vi "RT_VS50_Dynamics_DLR_v2.vi"() -> ()   [LabVIEW 2017]
uses:
  <vilib>/Platform/TimedLoop/XDataNode/timing_clust.ctl
  <vilib>/Platform/TimedLoop/XDataNode/nitl_modes.ctl
  <vilib>/Platform/TimedLoop/XDataNode/wakeup.ctl
  <vilib>/Analysis/coordinate.llb/Euler Rotation Order.ctl
  <vilib>/Analysis/baseanly.llb/Real A x B.vi
  <vilib>/Utility/file.llb/Read Delimited Spreadsheet (DBL).vi
  <vilib>/FPGAPlugInAG/Dynamic/niLvFpga_Close_Dynamic.vi
  <vilib>/Analysis/Matrix/Numeric/Conversions/Array To Matrix - RA2.vi
  <vilib>/Analysis/Matrix/Numeric/Conversions/Array To Matrix - RA.vi
  <vilib>/Analysis/Matrix/Numeric/Conversions/Matrix To Array - RM.vi
  <vilib>/platform/TimedLoop/XDataNode/XDataNode.xnode
  <vilib>/rvi/interface/nirviCloseFPGA/nirviCloseFPGA.xnode
  <vilib>/Platform/TimedLoop/XDataNode/XDNodeRunTimeDep.lvlib
  <vilib>/Analysis/Matrix/NI_Matrix.lvlib
  <vilib>/Analysis/NI_AALBase.lvlib
  <vilib>/Analysis/NI_AALPro.lvlib
panel:
  out "all rows":dbl[][](array[numeric]) format="%.9g"
  out "Math_OUT":dbl[](array[numeric])
  out "Velocity Mach":dbl
  out "latd(i) [º]":dbl
  out "lon(i) [º]":dbl
  out "acc_b":dbl[](array[numeric])
  out "SIM_Running 2":bool
  in  "Constant wind [m/s]":dbl format="%#_13g"
  out "Data 4":dbl[][](array[numeric])
  out "Data 3":dbl[][](array[numeric])
  in  "Wind_File":i32=1
  out "Data 2":dbl[][](array[numeric])
  out "TVA_Data CRC Fault":bool
  out "TVA_Address CRC Fault":bool
  out "Log":i64
  out "spreadsheet string":string
  in  "UTC format":bool
  out "appended path":path
  out "concatenated string":string
  out "SIM_Running":bool
  in  "stop RT":bool
  out "DMARS Write":i64
  out "TVA read":i64
  out "TVA_data":dbl[](array[numeric])
  out "bad iteration":bool
  out "Sim_Time":dbl
  out "string_DMARS":string
  out "lon(i) [rad]":dbl
  out "Euler Angles [rad]":dbl[](array[numeric])
  out "Euler Angles [º]":dbl[](array[numeric])
  out "M_beta":dbl
  out "M_alpha":dbl
  out "TVA_cmd [rad]":dbl[](array[numeric])
  out "Sref [m^2]":dbl
  out "MAd [Nm]":dbl[](array[numeric])
  out "MA_f [Nm]":dbl[](array[numeric])
  out "act_b":dbl[](array[numeric])
  out "p(i) [m]":dbl[](array[numeric])
  out "MFE_b":dbl[](array[numeric])
  out "alt(i) [m]":dbl
  out "latd(i) [rad]":dbl
  out "W_b(i) [º/s]":dbl[](array[numeric])
  out "q(i)":dbl[](array[numeric])
  out "W(i)":dbl[](array[numeric])
  out "V(i) [m/s]":dbl[](array[numeric])
  out "W(i+1)":dbl[](array[numeric])
  out "q(i+1)":dbl[](array[numeric])
  out "t [s]":dbl
  out "dt[s]":dbl
  out "ang_acc [rad/s^2]":dbl[](array[numeric])
  out "acc [m/s^2]":dbl[](array[numeric])
  out "MFA [Nm]":dbl[](array[numeric])
  out "MFE [Nm]":dbl[](array[numeric])
  out "Mco [Nm]":dbl[](array[numeric])
  out "Fco [N]":dbl[](array[numeric])
  out "FA [N]":dbl[](array[numeric])
  out "FG_b [N]":dbl[](array[numeric])
  out "FG [N]":dbl[](array[numeric])
  out "FE [N]":dbl[](array[numeric])
  out "FE_b [N]":dbl[](array[numeric])
  out "AoA_yaw [rad]":dbl
  out "AoA_pitch [rad]":dbl
  out "Iteration Duration [us]":i64(graph)
  out "Patm [Pa]":dbl
  out "Pdin [Pa]":dbl
  out "Nzl_S [m^2]":dbl
  out "Data":dbl[][](array[numeric])
  # "Time"
  # "TVA command"
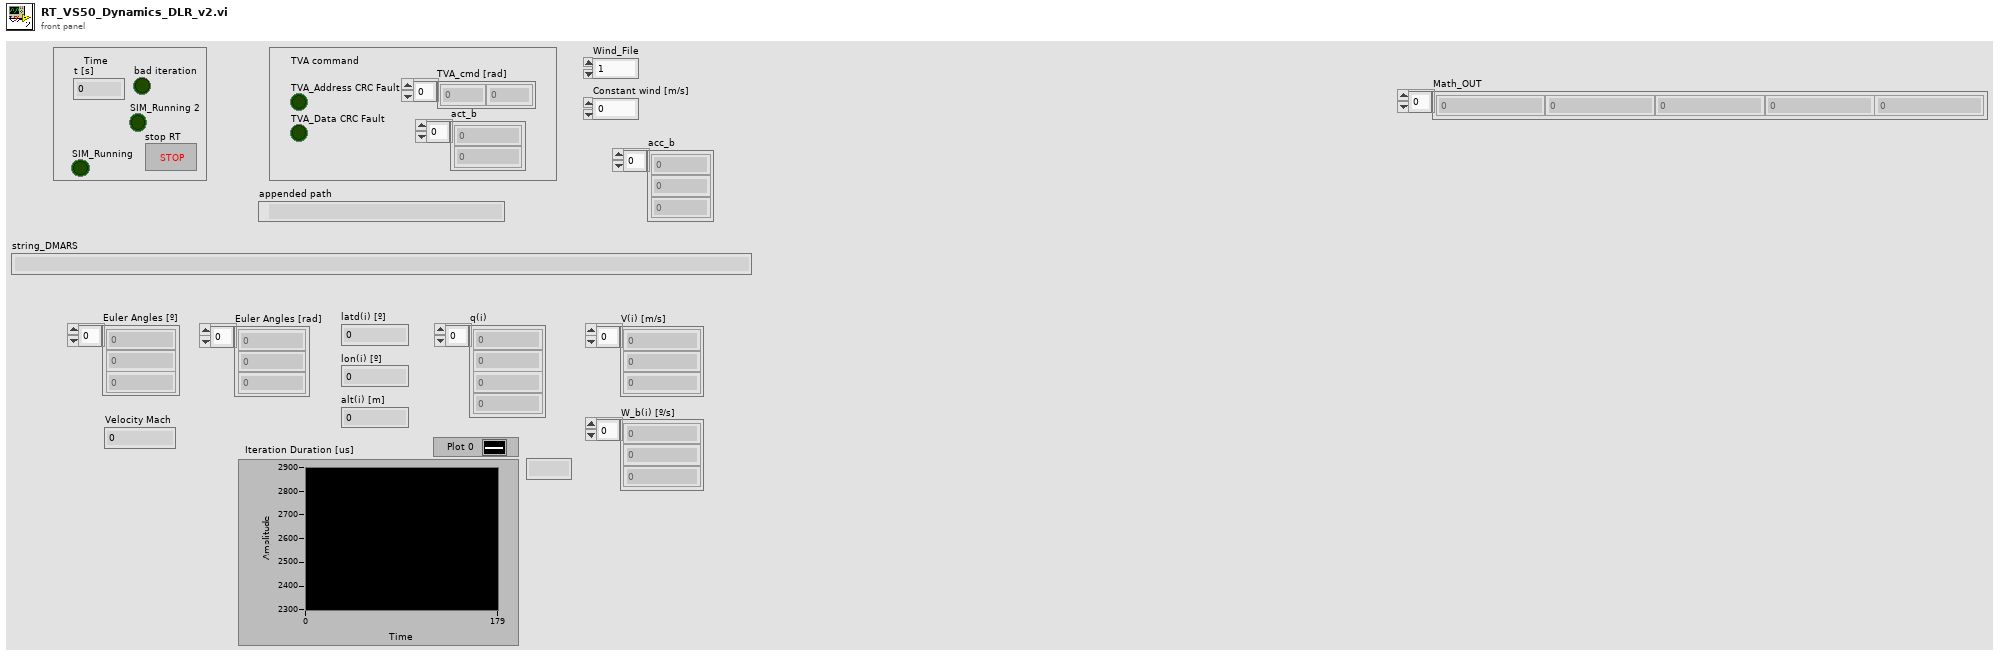
[diagram p1: front panel]
types:
  T1 = enum16{"open", "replace", "create", "open or create", "replace or create", "replace or create with confirmation"}
  T2 = typedef "XDNodeRunTimeDep.lvlib/timing_clust.ctl" = cluster{"Expected End [f-1]":u64, "Actual End [f-1]":u64, "Finished Late? [f-1]":bool, "Expected End [i-1]":u64, "Actual End [i-1]":u64, "Finished Late? [i-1]":bool, "Expected Start [i]":u64, "Actual Start [i]":u64, "Expected Start [f]":u64, "Actual Start [f]":u64, "Source Name":string, "Structure Name":string, "Period":i64, "Deadline":i64, "Offset":i64, "Start":i64, "Priority":i32, "Timeout":i32, "Mode":T3, "Wakeup Reason":T4, "Error":errorcluster, "Source Type":string, "Secondary Source Type":string, "Global End Time":u64, "Global Start Time":u64, "Frame Duration":u64, "Iteration Duration":u64, "Assigned CPU":i32, "I/O Scan Engine Mode":u32}
  T3 = typedef "XDNodeRunTimeDep.lvlib/nitl_modes.ctl" = enum32{"No Change", "Process missed periods, maintain original phase", "Discard missed periods, maintain original phase", "Process missed periods, ignore original phase", "Discard missed periods, ignore original phase"}
  T4 = typedef "XDNodeRunTimeDep.lvlib/wakeup.ctl" = enum32{"Normal", "Aborted", "Asynchronous wakeup", "Timing source error", "Timed loop error", "Timeout"}
  T5 = typedef "NI_AALPro.lvlib/Euler Rotation Order.ctl" = u16
  T6 = typedef "NI_Matrix.lvlib/RealMatrix.ctl" = dbl[][]
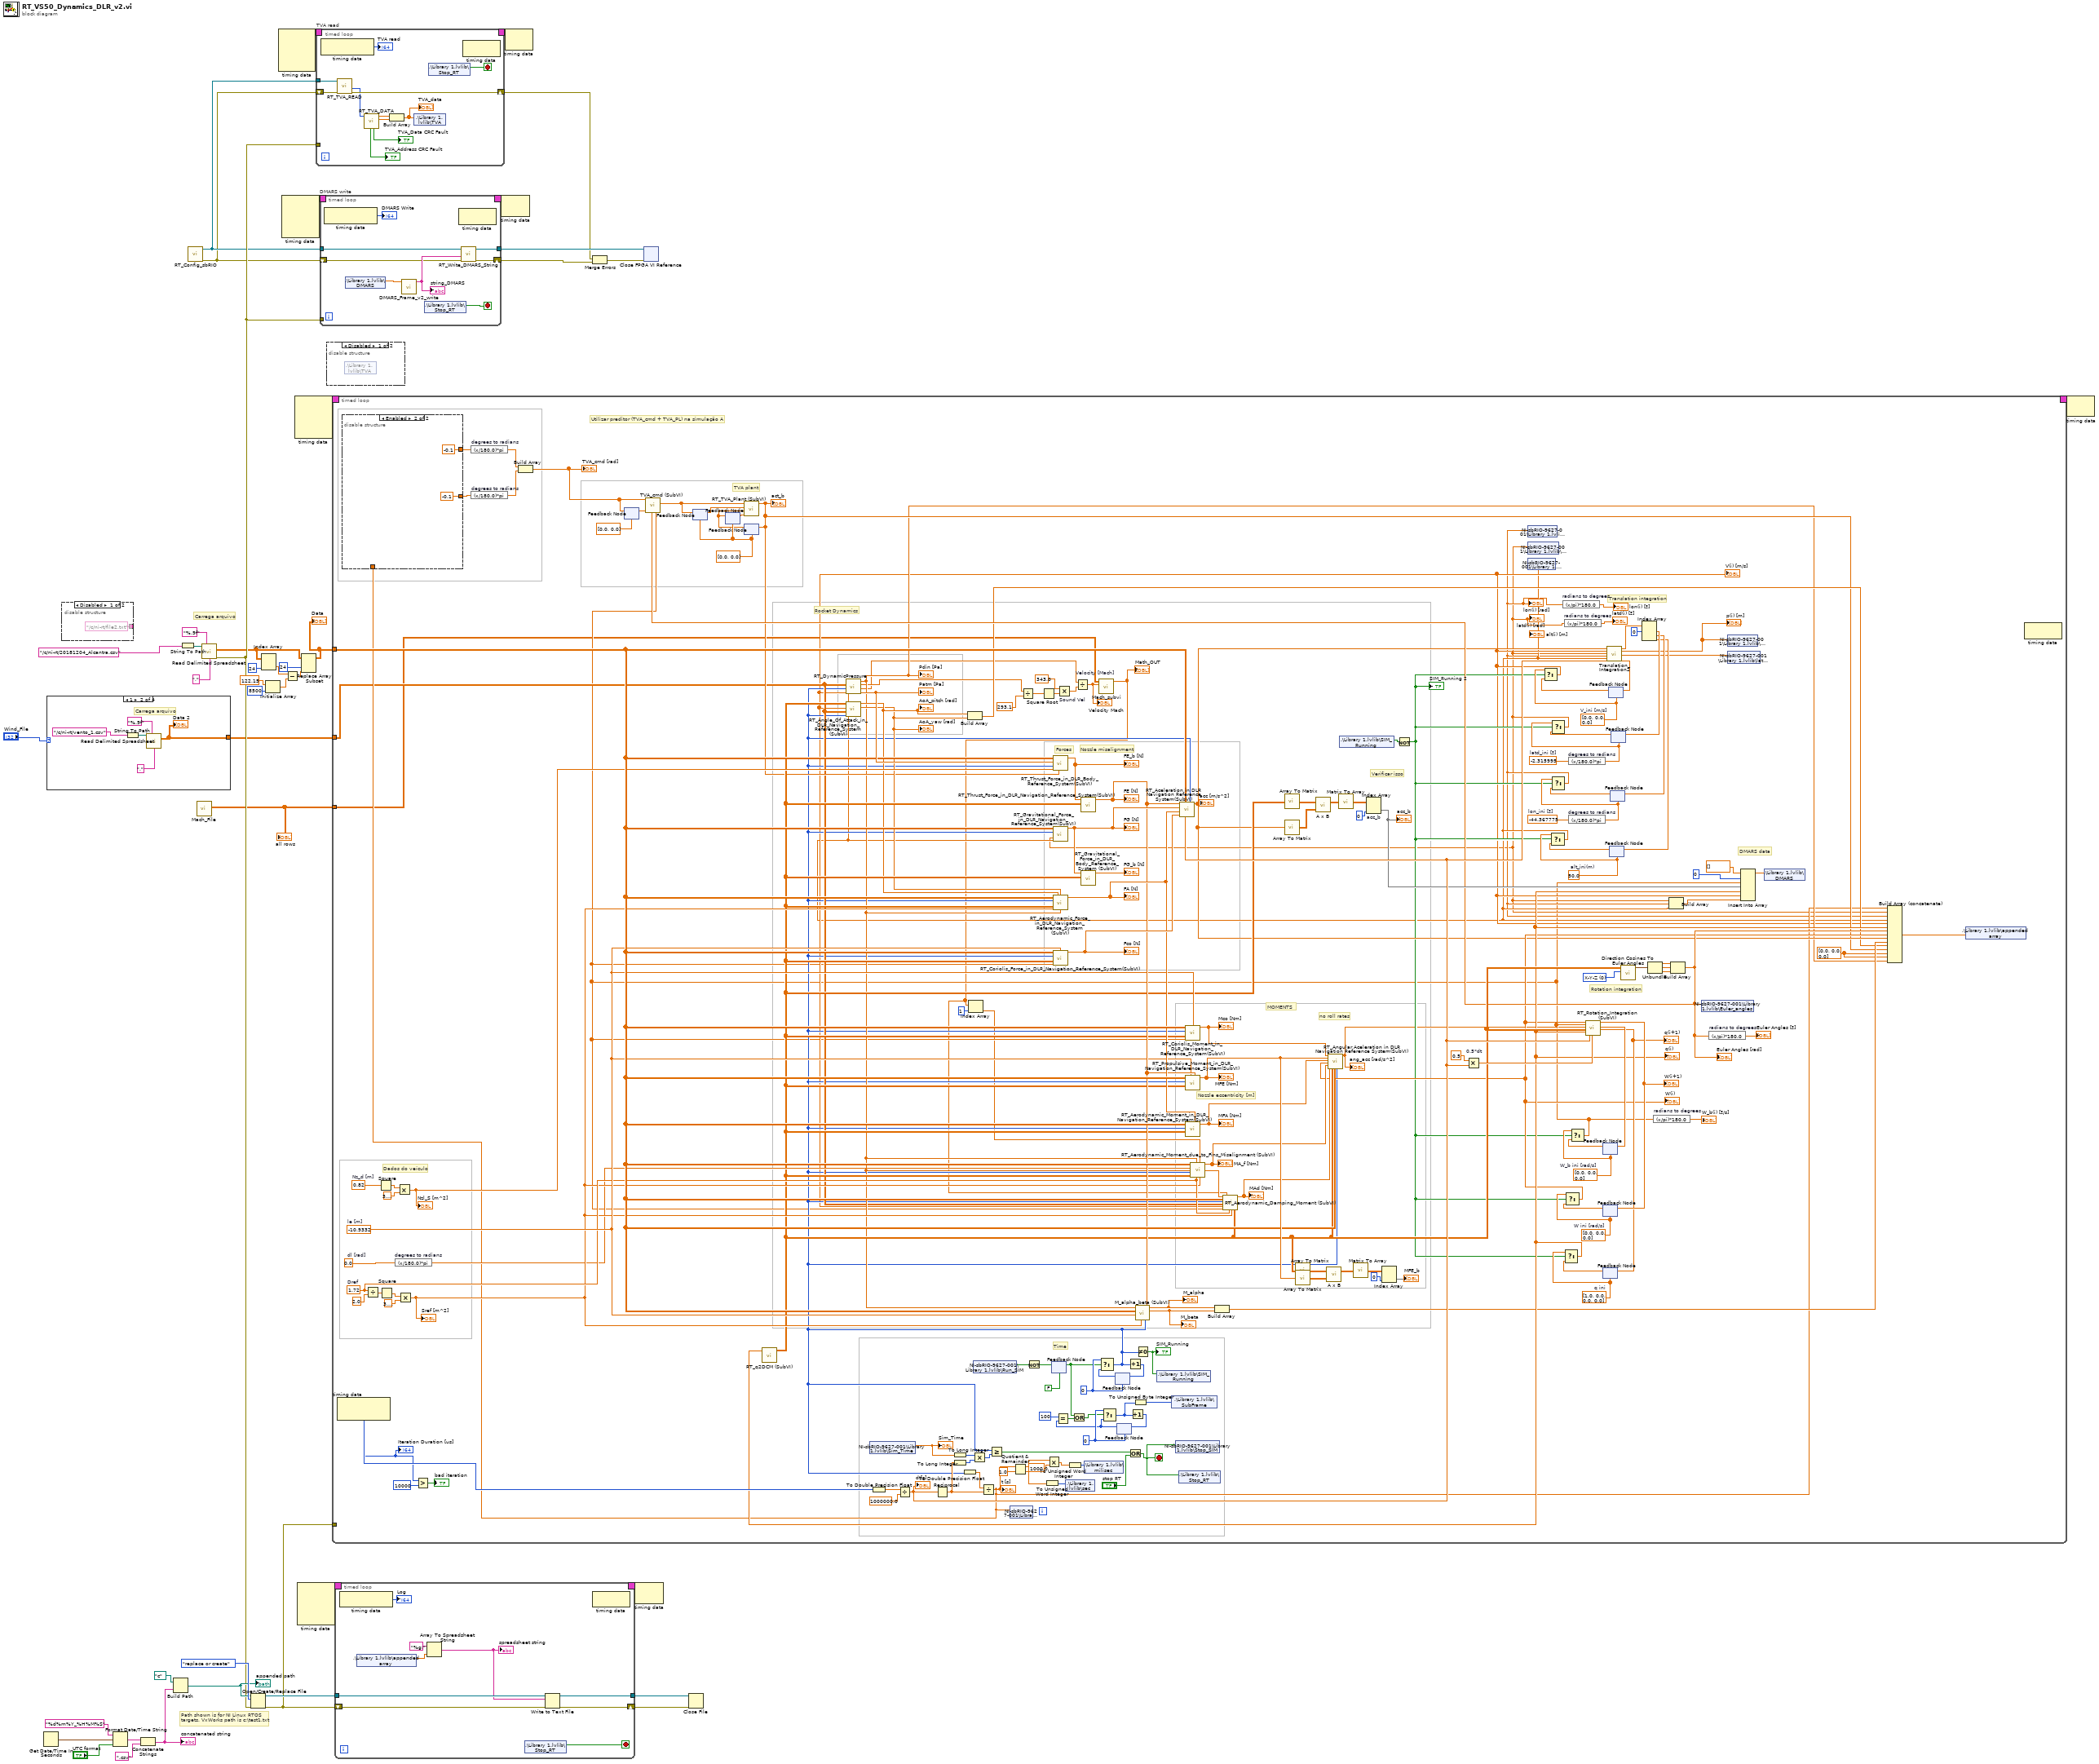
[diagram p0: block diagram]
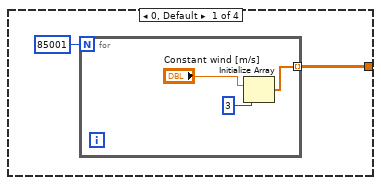
[diagram p4: hidden frame]
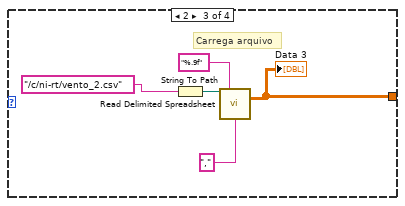
[diagram p5: hidden frame]
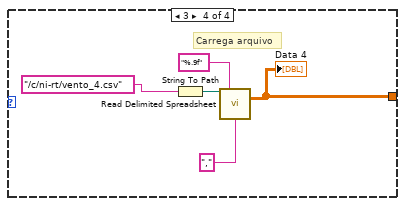
[diagram p6: hidden frame]
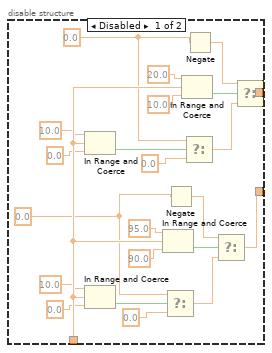
[diagram p7: hidden frame]
diagram:
  # "Path shown is for NI Linux RTOS\ntargets. VxWorks path is c:\\test1.txt"
  # "Carrega arquivo"
  n1 = Get Date/Time In Seconds() -> (seconds since 1Jan1904=w28:timestamp)
  n2 = case shown="1" "Wind_File" {
    tunnel: [w45 w50 w55 w60] -> w12
    frame 0, Default {
      n3 = for {
        N: 85001 -> [_]
        tunnel: [w47] -> w45 mode=indexing
        n4 = Initialize Array("Constant wind [m/s]", 3 ("dimension size")) -> (w47:dbl[])
      }
    }
    frame 1 {
      # "Carrega arquivo"
      n5 = String To Path(string="/c/ni-rt/vento_1.csv") -> (path=w52:path)
      n6 = call-poly <vilib>:"Read Delimited Spreadsheet.vi"("file path (dialog if empty)"=w52, "format (%.3f)"="%.9f", "delimiter (\\t)"="," ("delimiter (\\t)")) -> ("all rows"=w50:dbl[][])  [unwired: 7 in, 5 out]
      "Data 2" <- w50
    }
    frame 2 {
      # "Carrega arquivo"
      n7 = String To Path(string="/c/ni-rt/vento_2.csv") -> (path=w57:path)
      n8 = call-poly <vilib>:"Read Delimited Spreadsheet.vi"("file path (dialog if empty)"=w57, "format (%.3f)"="%.9f", "delimiter (\\t)"="," ("delimiter (\\t)")) -> ("all rows"=w55:dbl[][])  [unwired: 7 in, 5 out]
      "Data 3" <- w55
    }
    frame 3 {
      # "Carrega arquivo"
      n9 = String To Path(string="/c/ni-rt/vento_4.csv") -> (path=w62:path)
      n10 = call-poly <vilib>:"Read Delimited Spreadsheet.vi"("file path (dialog if empty)"=w62, "format (%.3f)"="%.9f", "delimiter (\\t)"="," ("delimiter (\\t)")) -> ("all rows"=w60:dbl[][])  [unwired: 7 in, 5 out]
      "Data 4" <- w60
    }
  }
  n11 = disable-structure shown="Disabled" {
    disable-tunnel: ["/c/ni-rt/file2.txt" _] -> _
    frame Disabled {
    }
    frame Enabled {
    }
  }
  n12 = Format Date/Time String(time format string (%c)="%d%m%Y_%H%M%S", seconds (now)=w28, UTC format="UTC format") -> (date/time string=w27:string)
  n13 = Concatenate Strings(w27, ".csv" ("string")) -> (w33:string)
  "concatenated string" <- w33
  n14 = Build Path(base path=path "c:/" ("file path (use dialog)"), name or relative path=w33) -> (appended path=w31:path)
  "appended path" <- w31
  n15 = String To Path(string="/c/ni-rt/20181204_Alcantra.csv") -> (path=w44:path)
  n16 = call "RT_Config_sbRIO.vi"() -> ("error out"=w17:errorcluster, "FPGA VI  Out"=w18:refnum<k20>)  [unwired: 10 in]
  n17 = call "Mach_File.vi"() -> ("all rows"=w1:dbl[][])  [unwired: 10 in, 1 out]
  "all rows" <- w1
  n18 = call-poly <vilib>:"Read Delimited Spreadsheet.vi"("file path (dialog if empty)"=w44, "format (%.3f)"="%.9f", "delimiter (\\t)"="," ("delimiter (\\t)")) -> ("all rows"=w3:dbl[][], "error out"=w25:errorcluster)  [unwired: 7 in, 4 out]
  n19 = Open/Create/Replace File(file path (use dialog)=w31, error in=w25, operation (0:open)=T1."replace or create") -> (refnum out=w36:refnum<file>, error out=w24:errorcluster)  [unwired: 3 in, 1 out]
  n20 = Index Array(array=w3, index (col)=24 ("disabled index (col)")) -> (element=w9:dbl[])  [unwired: 1 in]
  n21 = Initialize Array(122.15 ("element"), 8500 ("dimension size")) -> (w6:dbl[])
  n22 = node-c288() -> (w21:T2)  [unwired: 4 in]
  n23 = node-c288() -> (w23:T2)  [unwired: 4 in]
  n24 = Subtract(x=w9, y=w6) -> (x-y=w5:dbl[])
  n25 = node-c288() -> (w41:T2)  [unwired: 4 in]
  n26 = node-c288() -> (w39:T2)  [unwired: 4 in]
  n27 = Replace Array Subset(array=w3, new element=w5, index (col)=24 ("disabled index (col)")) -> (w2:dbl[][])  [unwired: 1 in]
  "Data" <- w2
  n28 = timed-loop "TVA read" {
    timing: w21 -> [_]
    timing-out: [_] -> w20
    tunnel: w18 -> [w76]
    shift-right: [w73] -> w15
    shift-left: w17 -> [w75]
    tunnel: w25 -> [_]
    stop <- w74 stop-if-true
    n29 = node-c288() -> (→"TVA read":i64)  [unwired: 1 in]
    n30 = call "RT_TVA_READ.vi"("error in (no error)"=w75, "FPGA VI  IN"=w76) -> ("error out"=w73:errorcluster, "Data"=w72:u64[])  [unwired: 7 in, 1 out]
    n31 = call "RT_TVA_DATA.vi"("TVA_Data"=w72) -> ("Yaw Angle"=w70:dbl, "Pitch Angle"=w71:dbl, "Data CRC Fault"=→"TVA_Data CRC Fault":bool, "Address CRC Fault"=→"TVA_Address CRC Fault":bool)  [unwired: 5 in, 2 out]
    n32 = Build Array(w71, w70) -> (w69:dbl[])
    "TVA_data" <- w69
    n33 = shared-variable ".\\Library 1.lvlib\\TVA"(w69) -> ()  [unwired: 1 in, 1 out]
    n34 = shared-variable ".\\Library 1.lvlib\\Stop_RT"() -> (w74:bool)  [unwired: 1 in, 1 out]
    n35 = node-c288() -> ()  [unwired: 1 in, 1 out]
  }
  n36 = timed-loop "DMARS write" {
    timing: w23 -> [_]
    timing-out: [_] -> w22
    tunnel: w25 -> [_]
    tunnel: w18 -> [w85]
    tunnel: [w83] -> w19
    shift-right: [w82] -> w14
    shift-left: w17 -> [w84]
    stop <- w87 stop-if-true
    n37 = node-c288() -> (→"DMARS Write":i64)  [unwired: 1 in]
    n38 = shared-variable ".\\Library 1.lvlib\\DMARS"() -> (w81:dbl[])  [unwired: 1 in, 1 out]
    n39 = call "DMARS_Frame_v2_write.vi"("DMARS"=w81) -> ("string_Out"=w86:string)  [unwired: 10 in]
    "string_DMARS" <- w86
    n40 = shared-variable ".\\Library 1.lvlib\\Stop_RT"() -> (w87:bool)  [unwired: 1 in, 1 out]
    n41 = node-c288() -> ()  [unwired: 1 in, 1 out]
    n42 = call "RT_Write_DMARS_String.vi"("error in (no error)"=w84, "String"=w86, "FPGA VI  IN"=w85) -> ("error out"=w82:errorcluster, "FPGA VI  Out"=w83:refnum<k20>)  [unwired: 7 in]
  }
  n43 = disable-structure shown="Disabled" {
    frame Disabled {
      n44 = shared-variable ".\\Library 1.lvlib\\TVA"() -> ()  [unwired: 1 in, 2 out]
    }
    frame Enabled {
    }
  }
  n45 = timed-loop {
    timing: w41 -> [_]
    timing-out: [_] -> w40
    tunnel: w2 -> [w234]
    tunnel: w24 -> [_]
    tunnel: w12 -> [w131]
    tunnel: w1 -> [w99]
    stop <- w142 stop-if-true
    w95 = dbl[] [0.0, 0.0] ("TVA_b")
    w217 = -44.367775  # lon_ini [º]
    w216 = -2.315995  # latd_ini [º]
    w123 = 0 ("x")
    w147 = dbl[] [0.0, 0.0, 0.0] ("array")
    w175 = 0 ("x")
    w189 = T5 0 items=["X-Y-Z", "X-Z-Y", "Y-X-Z", "Y-Z-X", "Z-X-Y", "Z-Y-X", "X-Y-X", "X-Z-X", "Y-X-Y", "Y-Z-Y", "Z-X-Z", "Z-Y-Z"] ("rotation order")
    w206 = 1.72  # Dref
    w195 = 0.0  # dl [rad]
    w211 = 0.82  # Nz_d [m]
    w207 = -10.9332  # le [m]
    w162 = dbl[] [0.0, 0.0, 0.0]  # W_b ini [rad/s]
    w168 = dbl[] [0.0, 0.0, 0.0]  # V_ini [m/s]
    w164 = 50.0  # alt_ini(m)
    w160 = dbl[] [0.0, 0.0, 0.0]  # W ini [rad/s]
    w158 = dbl[] [1.0, 0.0, 0.0, 0.0]  # q ini
    # "no roll rates"
    # "TVA plant"
    # "Nozzle eccentricity [m]"
    # "Nozzle misalignment"
    # "DMARS data"
    # "Rotation integration"
    # "Translation integration"
    # "Utilizar preditor (TVA_cmd + TVA_PL) na simulação A"
    # "Verificar isso"
    # "Rocket Dynamics"
    # "Time"
    # "Dados do veículo"
    # "MOMENTS"
    # "Forces"
    n46 = node-c288() -> (w193:i64, w254:i64)  [unwired: 1 in]
    "Iteration Duration [us]" <- w193
    n47 = Divide(x=w206, y=2.0) -> (x/y=w215:dbl)
    n48 = Square(x=w211) -> (x^2=w209:dbl)
    n49 = Square(x=w215) -> (x^2=w214:dbl)
    n50 = expression code="(x/180.0)*pi" "degrees to radians"(w195) -> (w194:dbl)
    n51 = Multiply(x=w209, y=3.141592653589793) -> (x*y=w208:dbl)
    "Nzl_S [m^2]" <- w208
    n52 = Multiply(x=w214, y=3.141592653589793) -> (x*y=w205:dbl)
    "Sref [m^2]" <- w205
    n53 = Greater?(x=w193, y=i64 10000) -> (0:→"bad iteration":bool)
    n54 = feedback #1(dbl[] [0.0, 0.0] ("TVA_cmd")) -> (w190:dbl[])
    n55 = feedback #2(w95) -> (w94:dbl[])
    n56 = feedback #3(w95) -> (w92:dbl[])
    n57 = feedback #4(w95) -> (w93:dbl[])
    n58 = feedback-in #3(w93) -> ()
    n59 = shared-variable "NI-sbRIO-9627-001\\Library 1.lvlib\\Sim_Time"() -> (w196:dbl)  [unwired: 1 in, 1 out]
    "Sim_Time" <- w196
    n60 = To Double Precision Float(number=w254) -> (double precision float=w253:dbl)
    n61 = Divide(x=w253, y=1000000.0) -> (x/y=w223:dbl)
    "dt[s]" <- w223
    n62 = Reciprocal(x=w223) -> (1/x=w250:dbl)
    n63 = To Long Integer(number=w196) -> (32bit integer=w197:i32)
    n64 = To Long Integer(number=w250) -> (32bit integer=w251:i32)
    n65 = Multiply(x=w197, y=w251) -> (x*y=w259:i32)
    n66 = shared-variable "NI-sbRIO-9627-001\\Library 1.lvlib\\Run_SIM"() -> (w172:bool)  [unwired: 1 in, 1 out]
    n67 = Not(x=w172) -> (.not. x?=w143:bool)
    n68 = feedback-in #5(w143) -> ()
    n69 = feedback #5(FALSE) -> (w120:bool)
    n70 = feedback #6(w175) -> (w174:i32)
    n71 = Select(t=w175, s=w120, f=w174) -> (s? t:f=w130:i32)
    n72 = To Double Precision Float(number=w130) -> (double precision float=w249:dbl)
    n73 = Divide(x=w249, y=w250) -> (x/y=w141:dbl)
    "t [s]" <- w141
    n74 = disable-structure shown="Enabled" {
      disable-tunnel: w141 -> [w282 _]
      disable-tunnel: [w279 -0.1 ("t")] -> w129
      disable-tunnel: [w260 -0.1 ("t")] -> w128
      frame Disabled {
        w261 = 0.0 ("TVA_y [º]")
        w272 = 0.0 ("TVA_p [º]")
        n75 = In Range and Coerce(upper limit=10.0, x=w282, lower limit=0.0) -> (In Range?=w277:bool)  [unwired: 1 out]
        n76 = In Range and Coerce(upper limit=10.0, x=w282, lower limit=0.0) -> (In Range?=w265:bool)  [unwired: 1 out]
        n77 = In Range and Coerce(upper limit=95.0, x=w282, lower limit=90.0) -> (In Range?=w264:bool)  [unwired: 1 out]
        n78 = Select(t=w261, s=w265, f=0.0 ("t")) -> (s? t:f=w263:dbl)
        n79 = Negate(x=w261) -> (-x=w262:dbl)
        n80 = In Range and Coerce(upper limit=20.0, x=w282, lower limit=10.0) -> (In Range?=w278:bool)  [unwired: 1 out]
        n81 = Select(t=w272, s=w277, f=0.0 ("t")) -> (s? t:f=w280:dbl)
        n82 = Negate(x=w272) -> (-x=w281:dbl)
        n83 = Select(t=w262, s=w264, f=w263) -> (s? t:f=w260:dbl)
        n84 = Select(t=w281, s=w278, f=w280) -> (s? t:f=w279:dbl)
      }
      frame Enabled {
      }
    }
    n85 = expression code="(x/180.0)*pi" "degrees to radians"(w129) -> (w127:dbl)
    n86 = expression code="(x/180.0)*pi" "degrees to radians"(w128) -> (w126:dbl)
    n87 = Build Array(w127, w126) -> (w132:dbl[])
    "TVA_cmd [rad]" <- w132
    n88 = feedback-in #1(w132) -> ()
    n89 = Greater Or Equal?(x=w130, y=w259) -> (x >= y?=w155:bool)
    n90 = shared-variable "NI-sbRIO-9627-001\\Library 1.lvlib\\t"(w141) -> ()  [unwired: 1 in, 1 out]
    n91 = Quotient & Remainder(x=w141, y=1.0) -> (x-y*floor(x/y)=w139:dbl, floor(x/y)=w135:dbl)
    n92 = To Unsigned Word Integer(number=w135) -> (unsigned 16bit integer=w134:u16)
    n93 = Multiply(x=w139, y=1000.0) -> (x*y=w137:dbl)
    n94 = shared-variable ".\\Library 1.lvlib\\sec"(w134) -> ()  [unwired: 1 in, 1 out]
    n95 = To Unsigned Word Integer(number=w137) -> (unsigned 16bit integer=w136:u16)
    n96 = shared-variable ".\\Library 1.lvlib\\milisec"(w136) -> ()  [unwired: 1 in, 1 out]
    n97 = feedback #7(w123) -> (w117:i32)
    n98 = Equal?(x=100, y=w117) -> (x = y?=w118:bool)
    n99 = Or(x=w120, y=w118) -> (x .or. y?=w119:bool)
    n100 = Select(t=w123, s=w119, f=w117) -> (s? t:f=w121:i32)
    n101 = Increment(x=w130) -> (x+1=w176:i32)
    n102 = feedback-in #6(w176) -> ()
    n103 = Or(x=w155, y="stop RT") -> (x .or. y?=w142:bool)
    n104 = Increment(x=w121) -> (x+1=w122:i32)
    n105 = feedback-in #7(w122) -> ()
    n106 = To Unsigned Byte Integer(number=w121) -> (unsigned 8bit integer=w133:u8)
    n107 = Not Equal To 0?(x=w130) -> (x != 0?=w157:bool)
    "SIM_Running" <- w157
    n108 = shared-variable ".\\Library 1.lvlib\\SIM_Running"(w157) -> ()  [unwired: 1 in, 1 out]
    n109 = shared-variable ".\\Library 1.lvlib\\SubFrame"(w133) -> ()  [unwired: 1 in, 1 out]
    n110 = shared-variable "NI-sbRIO-9627-001\\Library 1.lvlib\\Stop_SIM"(w142) -> ()  [unwired: 1 in, 1 out]
    n111 = shared-variable ".\\Library 1.lvlib\\Stop_RT"(w142) -> ()  [unwired: 1 in, 1 out]
    n112 = shared-variable ".\\Library 1.lvlib\\SIM_Running"() -> (w125:bool)  [unwired: 1 in, 1 out]
    n113 = Not(x=w125) -> (.not. x?=w124:bool)
    "SIM_Running 2" <- w124
    n114 = Multiply "0.5*dt"(x=0.5, y=w223) -> (x*y=w222:dbl)
    n115 = expression code="(x/180.0)*pi" "degrees to radians"(w216) -> (w170:dbl)
    n116 = expression code="(x/180.0)*pi" "degrees to radians"(w217) -> (w166:dbl)
    n117 = feedback #8(w160) -> (w161:dbl[])
    n118 = Select(t=w160, s=w124, f=w161) -> (s? t:f=w152:dbl[])
    "W(i)" <- w152
    n119 = feedback #9(w158) -> (w159:dbl[])
    n120 = Select(t=w158, s=w124, f=w159) -> (s? t:f=w154:dbl[])
    "q(i)" <- w154
    n121 = call "RT_q2DCM (SubVI).vi"("Quaternion"=w154) -> ("DCM"=w183:dbl[][])  [unwired: 10 in]
    n122 = call-poly <vilib>:"Array To Matrix.vi"("Real 2D Array"=w183) -> ("Real Matrix"=w204:T6)
    n123 = call-poly <vilib>:"Array To Matrix.vi"("Real 2D Array"=w183) -> ("Real Matrix"=w241:T6)
    n124 = feedback #10(w162) -> (w163:dbl[])
    n125 = Select(t=w162, s=w124, f=w163) -> (s? t:f=w108:dbl[])
    n126 = call "RT_Coriolis_Force_in_DLR_Navigation_Reference_System(SubVI).vi"("Data"=w234, "le (m) in"=w207, "i"=w130, "DCM"=w183, "W_b (rad/s)"=w108) -> ("Fco (N)"=w256:dbl[])  [unwired: 10 in]
    "Fco [N]" <- w256
    n127 = call "RT_Coriolis_Moment_in_DLR_Navigation_Reference_System(SubVI).vi"("Data"=w234, "le (m) in"=w207, "i"=w130, "DCM"=w183, "W_b (rad/s) in"=w108) -> ("Mco (Nm)"=w239:dbl[])  [unwired: 10 in]
    "Mco [Nm]" <- w239
    n128 = feedback #11(w168) -> (w169:dbl[])
    n129 = Select(t=w168, s=w124, f=w169) -> (s? t:f=w115:dbl[])
    "V(i) [m/s]" <- w115
    n130 = call "RT_Angle_Of_Attack_in_DLR_Navigation_Reference_System (SubVI).vi"("i"=w130, "V_wind [m/s]"=w131, "V (m/s)"=w115, "DCM"=w183) -> ("AoA_yaw (rad)"=w177:dbl, "AoA_pitch (rad)"=w178:dbl)  [unwired: 6 in]
    "AoA_pitch [rad]" <- w178
    "AoA_yaw [rad]" <- w177
    n131 = Build Array(w178, w177) -> (w149:dbl[])
    n132 = feedback #12(w164) -> (w165:dbl)
    n133 = Select(t=w164, s=w124, f=w165) -> (s? t:f=w114:dbl)
    "alt(i) [m]" <- w114
    n134 = call "RT_DynamicPressure.vi"("V (m/s)"=w115, "i"=w130, "V_wind [m/s]"=w131, "h (m)"=w114) -> ("Patm (Pa)"=w257:dbl, "air flow velocity [m/s]"=w101:dbl, "Temp [K]"=w102:dbl, "Pdin"=w146:dbl)  [unwired: 4 in]
    "Pdin [Pa]" <- w146
    "Patm [Pa]" <- w257
    n135 = Divide(x=w102, y=293.1) -> (x/y=w106:dbl)
    n136 = Square Root(x=w106) -> (sqrt(x)=w105:dbl)
    n137 = call "RT_Aerodynamic_Force_in_DLR_Navigation_Reference_System (SubVI).vi"("Data"=w234, "AoA_pitch (rad)"=w178, "AoA_yaw (rad)"=w177, "i"=w130, "DCM"=w183, "Sref [m^2]"=w205, "Pdin"=w146) -> ("FA"=w233:dbl[])  [unwired: 8 in]
    "FA [N]" <- w233
    n138 = Multiply "Sound Vel"(x=343.0, y=w105) -> (x*y=w103:dbl)
    n139 = Divide "Velocity [Mach]"(x=w101, y=w103) -> (x/y=w100:dbl)
    "Velocity Mach" <- w100
    n140 = call "Mach_subvi.vi"("Mach_IN"=w100, "Mach_File"=w99) -> ("OUT_Interp"=w96:dbl[])  [unwired: 9 in]
    "Math_OUT" <- w96
    n141 = Index Array(array=w96, index=1) -> (element=w97:dbl)
    n142 = call "RT_Aerodynamic_Moment_in_DLR_Navigation_Reference_System(SubVI).vi"("FA"=w233, "DCM"=w183, "i"=w130, "Data"=w234) -> ("MFA (Nm)"=w237:dbl[])  [unwired: 7 in]
    "MFA [Nm]" <- w237
    n143 = call "RT_Aerodynamic_Moment_due_to_Fins_Misalignment (SubVI).vi"("Sref [m^2]"=w205, "Cld 2"=w97, "Dref"=w206, "Pdin [Pa]"=w146, "DCM"=w183, "i"=w130, "dl [rad] in"=w194, "Data"=w234) -> ("MA_f"=w236:dbl[])  [unwired: 3 in]
    "MA_f [Nm]" <- w236
    n144 = call "RT_Aerodynamic_Damping_Moment (SubVI).vi"("Pdin [Pa]"=w146, "Data"=w234, "i"=w130, "V_wind [m/s]"=w131, "V(i) [m/s]"=w115, "W_b(i) [º/s]"=w108, "Mach coeficients"=w96, "Dref"=w206, "Sref [m^2]"=w205, "DCM"=w183) -> ("MAd"=w235:dbl[])  [unwired: 9 in]
    "MAd [Nm]" <- w235
    n145 = shared-variable "NI-sbRIO-9627-001\\Library 1.lvlib\\alt"(w114) -> ()  [unwired: 1 in, 1 out]
    n146 = feedback #13(w166) -> (w167:dbl)
    n147 = Select(t=w166, s=w124, f=w167) -> (s? t:f=w112:dbl)
    "lon(i) [rad]" <- w112
    n148 = shared-variable "NI-sbRIO-9627-001\\Library 1.lvlib\\lon"(w112) -> ()  [unwired: 1 in, 1 out]
    n149 = expression code="(x/pi)*180.0" "radians to degrees"(w112) -> (→"lon(i) [º]":dbl)
    n150 = feedback #14(w170) -> (w171:dbl)
    n151 = Select(t=w170, s=w124, f=w171) -> (s? t:f=w111:dbl)
    "latd(i) [rad]" <- w111
    n152 = call "RT_Gravitational_Force_in_DLR_Navigation_Reference_System(SubVI).vi"("Data"=w234, "i"=w130, "latd (rad)"=w111, "alt (m)"=w114) -> ("FG_d"=w255:dbl[])  [unwired: 10 in, 1 out]
    "FG [N]" <- w255
    n153 = call "RT_Gravitational_Force_in_DLR_Body_Reference_System (SubVI).vi"("DCM"=w183, "FG_d"=w255) -> ("FG_b"=→"FG_b [N]":dbl[])  [unwired: 9 in]
    n154 = shared-variable "NI-sbRIO-9627-001\\Library 1.lvlib\\latd"(w111) -> ()  [unwired: 1 in, 1 out]
    n155 = expression code="(x/pi)*180.0" "radians to degrees"(w111) -> (→"latd(i) [º]":dbl)
    n156 = call <vilib>:"Direction Cosines To Euler Angles.vi"("rotation order"=w189, "Direction Cosines"=w183) -> ("Euler Angles"=w186:cluster{"phi":dbl, "theta":dbl, "psi":dbl})  [unwired: 8 in, 1 out]
    n157 = Unbundle(w186) -> ("phi"=w188:dbl, "theta"=w187:dbl, "psi"=w185:dbl)
    n158 = expression code="(x/pi)*180.0" "radians to degrees"(w108) -> (→"W_b(i) [º/s]":dbl[])
    n159 = Build Array(w111, w112, w114) -> (w113:dbl[])
    n160 = Build Array(w188, w187, w185) -> (w153:dbl[])
    "Euler Angles [rad]" <- w153
    n161 = call "TVA_cmd (SubVI).vi"("W_b [rad/s]"=w108, "Angles [rad]"=w153, "TVA_old [rad]"=w190, "TVA_cmd [rad]"=w132) -> ("Act315_Act225"=w184:dbl[])  [unwired: 6 in, 1 out]
    n162 = feedback-in #2(w184) -> ()
    n163 = call "RT_TVA_Plant (SubVI).vi"("TVA_b(i-2)"=w92, "TVA_b(i-1)"=w93, "TVA_cmd (i-2) [rad]"=w94, "TVA_cmd (i-1) [rad]"=w184) -> ("TVA_b"=w148:dbl[])  [unwired: 7 in]
    "act_b" <- w148
    n164 = feedback-in #4(w148) -> ()
    n165 = call "RT_Thrust_Force_in_DLR_Body_Reference_System(SubVI).vi"("Act_b(i)"=w148, "Nzl_S"=w208, "i"=w130, "Patm (Pa)"=w257, "Data"=w234) -> ("FE_b"=w247:dbl[])  [unwired: 6 in]
    "FE_b [N]" <- w247
    n166 = call "RT_Thrust_Force_in_DLR_Navigation_Reference_System(SubVI).vi"("DCM"=w183, "FE_b"=w247) -> ("FE"=w232:dbl[])  [unwired: 8 in]
    "FE [N]" <- w232
    n167 = call "M_alpha_beta (SubVI).vi"("i"=w130, "Sref"=w205, "FE [N]"=w232, "le [m]"=w207, "Data"=w234, "Pdin [Pa]"=w146) -> ("M_beta"=w179:dbl, "M_alpha"=w180:dbl)  [unwired: 4 in]
    "M_alpha" <- w180
    "M_beta" <- w179
    n168 = call "RT_Aceleration in DLR Navigation Reference System(SubVI).vi"("i"=w130, "dt(s)"=w223, "Data"=w234, "Fco (N)"=w256, "FA"=w233, "FG"=w255, "FE"=w232) -> ("acc"=w151:dbl[])  [unwired: 4 in]
    "acc [m/s^2]" <- w151
    n169 = call "RT_Propulsive_Moment_in_DLR_Navigation_Reference_System(SubVI).vi"("FE"=w232, "le (m) in"=w207, "DCM"=w183, "i"=w130, "Data"=w234) -> ("MFE (Nm)"=w238:dbl[])  [unwired: 6 in]
    "MFE [Nm]" <- w238
    n170 = Build Array(w180, w179) -> (w150:dbl[])
    n171 = call-poly <vilib>:"Array To Matrix.vi"("Real 1D Array"=w151) -> ("Real Matrix (Column Vector)"=w203:T6)
    n172 = call-poly <vilib>:"Array To Matrix.vi"("Real 1D Array"=w238) -> ("Real Matrix (Column Vector)"=w246:T6)
    n173 = call-poly <vilib>:"A x B.vi"("B"=w203, "A"=w204) -> ("A x B"=w201:T6)  [unwired: 1 out]
    n174 = call-poly <vilib>:"A x B.vi"("B"=w246, "A"=w241) -> ("A x B"=w244:T6)  [unwired: 1 out]
    n175 = call "RT_Angular Aceleration in DLR Navigation Reference System(SubVI).vi"("Mco (Nm)"=w239, "MFE (Nm)"=w238, "MFA (Nm)"=w237, "W (rad/s)"=w152, "MA_f [Nm]"=w236, "MAd [Nm]"=w235, "DCM"=w183, "Data"=w234, "i"=w130) -> ("ang_acc"=w91:dbl[])  [unwired: 10 in]
    "ang_acc [rad/s^2]" <- w91
    n176 = call-poly <vilib>:"Matrix To Array.vi"("Real Matrix"=w201) -> ("Real 2D Array"=w202:dbl[][])
    n177 = call-poly <vilib>:"Matrix To Array.vi"("Real Matrix"=w244) -> ("Real 2D Array"=w245:dbl[][])
    n178 = Index Array "acc_b"(array=w202, index (col)=0 ("index (row)")) -> (element=w181:dbl[])  [unwired: 1 in]
    "acc_b" <- w181
    n179 = Index Array(array=w245, index (col)=0 ("index (row)")) -> (element=→"MFE_b":dbl[])  [unwired: 1 in]
    n180 = call "RT_Rotation_Integration (SubVI).vi"("W(i) [rad/s] in"=w152, "W_b(i) [rad/s]"=w108, "ang_acc [rad/s^2]"=w91, "D_NB"=w183, "q(i) in"=w154, "dt"=w223, "dt*0.5"=w222) -> ("W(i+1)"=w221:dbl[], "W_b(i+1) [rad/s]"=w220:dbl[], "q(i+1)"=w219:dbl[])  [unwired: 9 in, 1 out]
    "q(i+1)" <- w219
    "W(i+1)" <- w221
    n181 = feedback-in #8(w221) -> ()
    n182 = feedback-in #9(w219) -> ()
    n183 = feedback-in #10(w220) -> ()
    n184 = call "Translation_Integration2.vi"("acc"=w151, "V(i) in"=w115, "latd(i)"=w111, "lon(i) [rad]"=w112, "alt(i) [m]"=w114, "dt [s]"=w223) -> ("position"=w182:dbl[], "position ECEF (i)"=w224:dbl[], "L_C"=w225:dbl, "Velocity"=w226:dbl[])  [unwired: 10 in]
    "p(i) [m]" <- w224
    n185 = feedback-in #11(w226) -> ()
    n186 = Index Array(array=w182, index #1=0 ("index")) -> (element #1=w229:dbl, element #2=w228:dbl, element #3=w227:dbl)  [unwired: 2 in]
    n187 = feedback-in #12(w227) -> ()
    n188 = feedback-in #13(w228) -> ()
    n189 = feedback-in #14(w229) -> ()
    n190 = shared-variable "NI-sbRIO-9627-001\\Library 1.lvlib\\Euler_angles"(w153) -> ()  [unwired: 1 in, 1 out]
    n191 = expression code="(x/pi)*180.0" "radians to degrees"(w153) -> (→"Euler Angles [º]":dbl[])
    n192 = shared-variable "NI-sbRIO-9627-001\\Library 1.lvlib\\Pos"(w224) -> ()  [unwired: 1 in, 1 out]
    n193 = shared-variable "NI-sbRIO-9627-001\\Library 1.lvlib\\lat_c"(w225) -> ()  [unwired: 1 in, 1 out]
    n194 = Insert Into Array(array=dbl[] [], index=0, new element #1=w108, new element #2=w181, new element #3=w154, new element #4=w115, new element #5=w113) -> (w144:dbl[])
    n195 = shared-variable ".\\Library 1.lvlib\\DMARS"(w144) -> ()  [unwired: 1 in, 1 out]
    n196 = Build Array (concatenate)(w141, w111, w112, w114, w115, w154, w153, w152, w151, w150, w149, w148, w147, w147, w146) -> (w145:dbl[])
    n197 = shared-variable ".\\Library 1.lvlib\\appended array"(w145) -> ()  [unwired: 1 in, 1 out]
    n198 = node-c288() -> ()  [unwired: 1 in, 1 out]
  }
  n199 = timed-loop {
    tunnel: w36 -> [w297]
    tunnel: [w296] -> w35
    timing: w39 -> [_]
    timing-out: [_] -> w38
    shift-right: [w289] -> w26
    shift-left: w24 -> [w290]
    stop <- w295 stop-if-true
    n200 = node-c288() -> (→"Log":i64)  [unwired: 1 in]
    n201 = shared-variable ".\\Library 1.lvlib\\appended array"() -> (w292:dbl[])  [unwired: 1 in, 1 out]
    n202 = Array To Spreadsheet String(array=w292, 3:"%g;" ("format string")) -> (spreadsheet string=w291:string)  [unwired: 1 in]
    "spreadsheet string" <- w291
    n203 = shared-variable ".\\Library 1.lvlib\\Stop_RT"() -> (w295:bool)  [unwired: 1 in, 1 out]
    n204 = Write to Text File(file (use dialog)=w297, text=w291, error in=w290) -> (refnum out=w296:refnum<file>, error out=w289:errorcluster)  [unwired: 1 in, 1 out]
    n205 = node-c288() -> ()  [unwired: 1 in, 1 out]
  }
  n206 = node-c288(w22) -> ()  [unwired: 1 out]
  n207 = node-c288(w20) -> ()  [unwired: 1 out]
  n208 = Merge Errors(w15, w14) -> (w16:errorcluster)
  n209 = node-c288(w38) -> ()  [unwired: 1 out]
  n210 = xnode "Close FPGA VI Reference"("FPGA VI Reference In"=w19, "error in"=w16) -> ()  [unwired: 1 out]
  n211 = Close File(refnum=w35, error in=w26) -> ()  [unwired: 2 out]
  n212 = node-c288(w40) -> ()  [unwired: 1 out]
